vi "Set Tools Splitter position.vi"(9 "Show":bool=TRUE, 10 "Splitter Tools":refnum<vi>, 11 "VI in":refnum<vi>) -> (0 "error out":errorcluster)   [LabVIEW 2019, in "Panther Dashboard.lvlib"]
uses:
  Panther Dashboard.lvlib
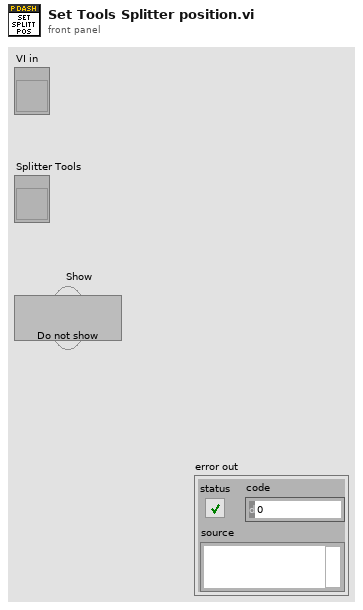
[diagram p1: front panel]
types:
  T1 = typedef "LVRectTypeDef.ctl" = cluster{"Left":i16, "Top":i16, "Right":i16, "Bottom":i16}
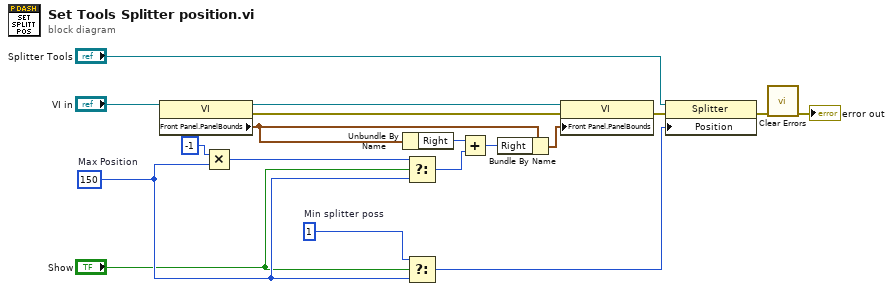
[diagram p0: block diagram]
diagram:
  w10 = 1  # Min splitter poss
  w8 = 150  # Max Position
  n1 = property class="VI"(reference="VI in") -> (reference out=w1:refnum<vi>, error out=w17:errorcluster, "Front Panel.PanelBounds"=w2:T1)  [unwired: 1 in]
  n2 = Multiply(x=-1, y=w8) -> (x*y=w9:i32)
  n3 = Unbundle By Name(w2) -> ("Right"=w4:i16)
  n4 = Select(t=w9, s="Show", f=w8) -> (s? t:f=w14:i32)
  n5 = Select(t=w10, s="Show", f=w8) -> (s? t:f=w12:i32)
  n6 = Add(x=w4, y=w14) -> (x+y=w5:i32)
  n7 = Bundle By Name(cluster=w2, "Right"=w5) -> (w3:T1)
  n8 = property class="VI"(reference=w1, error in=w17, "Front Panel.PanelBounds"=w3) -> (error out=w16:errorcluster)  [unwired: 1 out]
  n9 = property class="Splitter"(reference="Splitter Tools", error in=w16, "Position"=w12) -> (error out=w15:errorcluster)  [unwired: 1 out]
  n10 = call <vilib>:"Clear Errors.vi"("error in (no error)"=w15) -> ("error out"=→"error out":errorcluster)  [unwired: 5 in, 1 out]
